vi "PH-temp.vi"(2 "ltstream in":u16[][](array[numeric]), 3 "pstream in":u16[](array[numeric]), 4 "String":string) -> (0 "ltstream out":u16[][](array[numeric]), 1 "pstream out":u16[](array[numeric]))   [LabVIEW 2015]
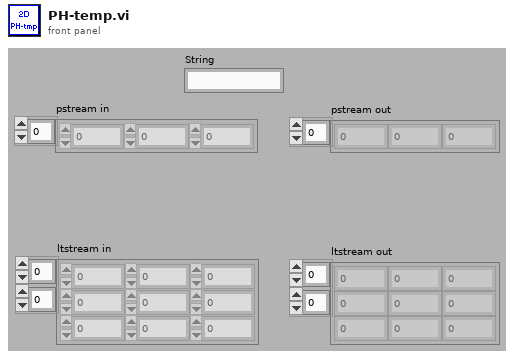
[diagram p1: front panel]
types:
  T1 = cluster{"initialized":bool, "devidx":i32, "Ch0 Level":i32, "Ch0 ZeroX":i32, "Ch1 Level":i32, "Ch1 ZeroX":i32, "sync rate":i32, "resolution":i32, "acq time":i32, "acq rate":i32, "# bins":u32, "Bin size":enum16{"1", "2", "4", "8", "16", "32", "64", "128"}, "min photons":u32, "truncate":u32}
  T2 = typedef "LVRectTypeDef.ctl" = cluster{"Left":i16, "Top":i16, "Right":i16, "Bottom":i16}
  T3 = cluster{"Xpixels":i32, "Vxminref":dbl, "Vxmaxref":dbl, "P":dbl, "Ypixels":i32, "Vyminref":dbl, "Vymaxref":dbl, "srate":sgl, "sAOxy":i32, "timeout":dbl, "type":string, "date":string, "time":string, "Colormap":u16, "Drawing Mode":u16, "Scanning Mode":u16, "square pixels":bool, "square matrix":bool, "Xpixels Img":i32, "Vx-min Img":dbl, "VX-max Img":dbl, "Ypixels Img":i32, "Vy-min Img":dbl, "Vy-max Img ":dbl, "Angle Img":dbl, "autoshutter":bool, "finite":bool, "cont":bool, "wavdet":bool, "measpoints":i32, "avpp":i32, "bufferAO":i32, "bufferAI":i32, "starttick":u32, "waveform":path, "Vx-ref":dbl, "Vy-ref":dbl, "refreshrate":dbl, "refreshbuffer":i32, "tt_cycles":i32, "motorref":refnum<k7>, "mirrorswitch":refnum<k7>, "sample mode":i32, "maxbufferAI":i32, "srateAODO":sgl, "bin":sgl, "Pel":sgl, "Angle draw":dbl, "srate Img":sgl, "ROIimg_plotbounds":T2, "auto OD":bool, "ODfilt":u16, "aAI":i32[], "aCI":i32[], "aAO":u32[], "aDO":u32[], "refwfsize":dbl, "Lifetime":bool, "Vz-Img":dbl, "Vz-ref":dbl, "Vz-reset":dbl, "AIoverride":bool, "aAS":u32[], "XYZstart":dbl[], "External 100KHz Clock?":bool}
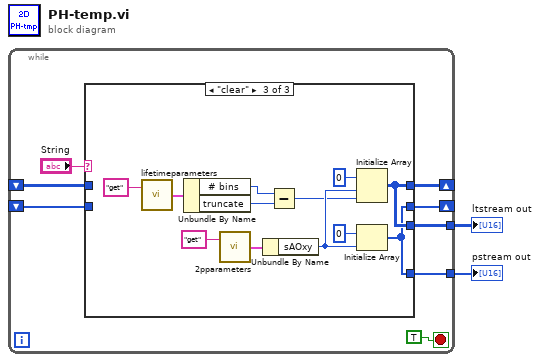
[diagram p0: block diagram]
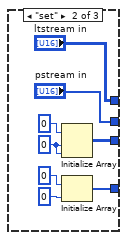
[diagram p3: hidden frame]
diagram:
  n1 = while {
    shift-right: [w9] -> _
    shift-left: _ -> [w10]
    tunnel: [w8] -> w2
    shift-right: [w5] -> _
    shift-left: _ -> [w3]
    tunnel: [w4] -> w1
    stop <- TRUE stop-if-true
    n2 = case shown="\"clear\"" "String" {
      tunnel: [w12 "ltstream in" w31] -> w9
      tunnel: w10 -> [w12 _ _]
      tunnel: [w12 w19 w31] -> w8
      tunnel: [w11 "pstream in" w29] -> w5
      tunnel: [w11 w13 w29] -> w4
      tunnel: w3 -> [w11 _ _]
      frame "get", Default {
      }
      frame "set" {
        w18 = 0 ("dimension size")
        n3 = Initialize Array(u16 0 ("element"), w18, w18) -> (w19:u16[][])
        n4 = Initialize Array(u16 0 ("element"), 0 ("dimension size")) -> (w13:u16[])
      }
      frame "clear" {
        n5 = call "lifetimeparameters.vi"("command"="get") -> ("Params out"=w24:T1)  [unwired: 1 in]
        n6 = Unbundle By Name(w24) -> ("# bins"=w23:u32, "truncate"=w22:u32)
        n7 = call "2pparameters.vi"("command"="get") -> ("params out"=w27:T3)  [unwired: 1 in]
        n8 = Unbundle By Name(w27) -> ("sAOxy"=w26:i32)
        n9 = Subtract(x=w23, y=w22) -> (x-y=w21:u32)
        n10 = Initialize Array(u16 0 ("element"), w26, w21) -> (w31:u16[][])
        n11 = Initialize Array(u16 0 ("element"), w26) -> (w29:u16[])
      }
    }
  }
  "pstream out" <- w1
  "ltstream out" <- w2
